vi "C3.vi"(8 "Error":errorcluster, 11 "KNR in":T1) -> (0 "error out":errorcluster, 1 "Number of Matches (Shape Detection 1)":i32, 2 "Circles (Shape Detection 1)":T3(array[cluster]) {"Position"."Y" format="%.2f"; "Position"."X" format="%.2f"}, 3 "KNR out 4":T1, 5 "Image Out":T4)   [LabVIEW 2013]
uses:
  <vilib>/vision/Image Controls.llb/IMAQ Image.ctl
  <userlib>/KNR OS 3.0 LabVIEW Toolkit/Type Definition/KNR3 Reference.ctl
  <userlib>/_FPGA Interface Advanced Tools/FPGA Interface Base/FPGA Interface Base.lvclass
  <userlib>/KNR OS 3.0 LabVIEW Toolkit/Type Definition/Resource.ctl
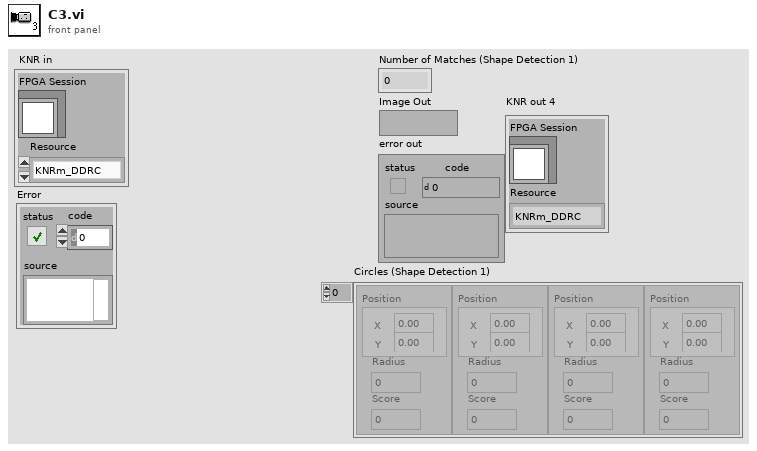
[diagram p1: front panel]
types:
  T1 = typedef "KNR3 Reference.ctl" = cluster{"FPGA Session":refnum<class "FPGA Interface Base.lvclass">, "Resource":T2}
  T2 = typedef "Resource.ctl" = enum16{"KNRm_DDRC", "KNRm_DDDD", "KNRm_DDDR", "KNRm_DDDC", "KNR"}
  T3 = cluster{"Position":cluster{"X":sgl, "Y":sgl}, "Radius":dbl, "Score":dbl}[]
  T4 = typedef "IMAQ Image.ctl" = refnum<image>
  T5 = cluster{"Mode":enum16{"FRWD", "TURFIX", "TURNOF", "CIRCULAR"}, "Dir":enum16{"Left", "Right"}, "Pcmd":dbl, "Vcmd":dbl, "X":dbl, "Y":dbl}
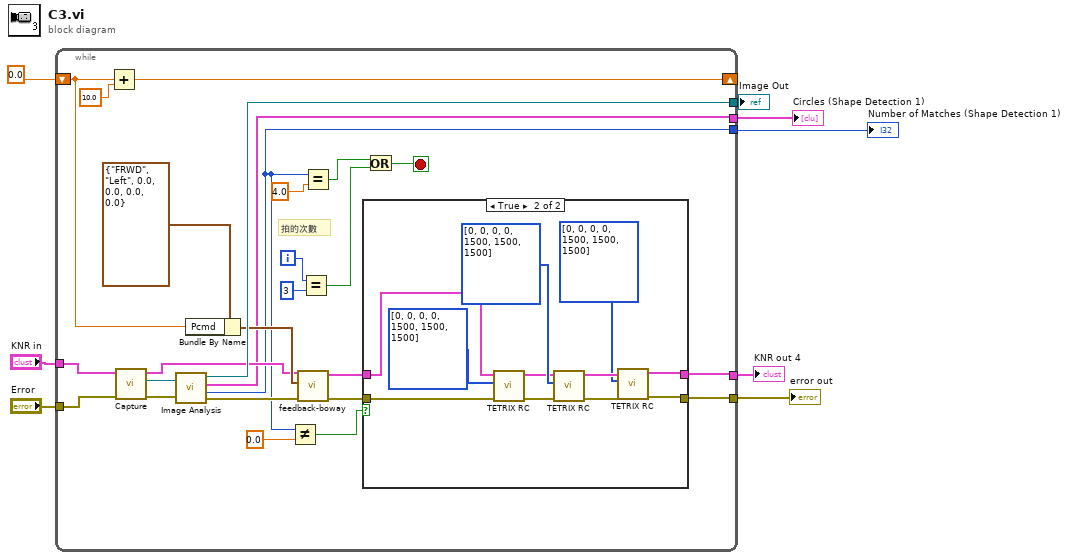
[diagram p0: block diagram]
diagram:
  n1 = while {
    tunnel: [w11] -> w8
    tunnel: [w33] -> w7
    tunnel: "KNR in" -> [w32]
    tunnel: "Error" -> [w31]
    tunnel: [w19] -> w4
    shift-right: [w27] -> _
    shift-left: 0.0 -> [w26]
    tunnel: [w22] -> w2
    tunnel: [w18] -> w1
    i -> [w16]
    stop <- w14 stop-if-true
    # "拍的次數"
    n2 = Add(x=w26, y=10.0) -> (x+y=w27:dbl)
    n3 = call "Capture.vi"("Error"=w31, "KNR in"=w32) -> ("error out"=w30:errorcluster, "Image Out"=w34:T4, "KNR out"=w23:T1)  [unwired: 7 in]
    n4 = call "Image Analysis.vi"("Image In"=w34, "error in"=w30) -> ("Image Out"=w33:T4, "Circles (Shape Detection 1)"=w22:T3, "Number of Matches (Shape Detection 1)"=w11:i32, "error out"=w29:errorcluster)
    n5 = Bundle By Name(cluster=T5 {"Mode"=enum."FRWD", "Dir"=enum."Left", "Pcmd"=0.0, "Vcmd"=0.0, "X"=0.0, "Y"=0.0} ("Move"), "Pcmd"=w26) -> (w25:T5)
    n6 = Not Equal?(x=w11, y=0.0) -> (x != y?=w9:bool)
    n7 = call "feedback-boway.vi"("error in (no error)"=w29, "Move"=w25, "KNR in"=w23) -> ("error out"=w21:errorcluster, "KNR out"=w20:T1)  [unwired: 6 in, 1 out]
    n8 = Equal?(x=w16, y=3) -> (x = y?=w12:bool)
    n9 = Equal?(x=w11, y=4.0) -> (x = y?=w13:bool)
    n10 = case shown="True" w9 {
      tunnel: w21 -> [w35 w47]
      tunnel: w20 -> [w36 w43]
      tunnel: [w35 w38] -> w19
      tunnel: [w36 w39] -> w18
      frame False {
      }
      frame True {
        n11 = call "TETRIX RC.vi"("error in 2"=w47, "RC"=u16[] [0, 0, 0, 0, 1500, 1500, 1500], "KNR in 3"=w43) -> ("error out 4"=w46:errorcluster, "KNR out 4"=w42:T1)  [unwired: 7 in]
        n12 = call "TETRIX RC.vi"("error in 2"=w46, "RC"=u16[] [0, 0, 0, 0, 1500, 1500, 1500], "KNR in 3"=w42) -> ("error out 4"=w41:errorcluster, "KNR out 4"=w40:T1)  [unwired: 7 in]
        n13 = call "TETRIX RC.vi"("error in 2"=w41, "RC"=u16[] [0, 0, 0, 0, 1500, 1500, 1500], "KNR in 3"=w40) -> ("error out 4"=w38:errorcluster, "KNR out 4"=w39:T1)  [unwired: 7 in]
      }
    }
    n14 = Or(x=w13, y=w12) -> (x .or. y?=w14:bool)
  }
  "Number of Matches (Shape Detection 1)" <- w8
  "Image Out" <- w7
  "error out" <- w4
  "Circles (Shape Detection 1)" <- w2
  "KNR out 4" <- w1
